vi "Begin.vi"(8 "error in":errorcluster) -> (0 "error out":errorcluster)   [LabVIEW 2018]
doc: "Called before other user functions, this VI is expected to open initial I/O refnums, load in file data, and do all program initialization. Notice that the <B>error out</B> terminal is simply used for data flow. Wiring it to other structures or subVIs ensures that this VI runs first."
uses:
  <vilib>/Rock Robotics/SystemInterfaces/DIO/FPGA_DIOPWMChannel.ctl
  <vilib>/Rock Robotics/WPI/DriverStation/WPI_DriverStationRobotMode2.ctl
  <vilib>/Rock Robotics/WPI/Joystick/WPI_JoystickDeviceEnum.ctl
  <vilib>/Rock Robotics/WPI/Solenoid/WPI_SolenoidChannel.ctl
  <vilib>/Rock Robotics/SystemInterfaces/DIO/FPGA_DIOChannel.ctl
  <vilib>/Rock Robotics/WPI/SafetyOutput/WPI_SafetyOutputConfigMenu.ctl
  Robot Global Data.vi
  <vilib>/Rock Robotics/Network Tables/NT Write String Array.vi
  <vilib>/Rock Robotics/WPI/RobotDrive/WPI_RobotDriveOpen4MotorWithTalonSRX.vi
  <vilib>/Rock Robotics/WPI/Switch/WPI_SwitchOpenLimit.vi
  <vilib>/Rock Robotics/WPI/MotorControl/WPI_MotorControlOpen TalonSRX.vi
  Global 1.vi
  <vilib>/Rock Robotics/WPI/Counter/WPI_CounterDigitalInputToDigitalSource.vi
  <vilib>/Rock Robotics/WPI/Solenoid/WPI_SolenoidOpenDouble.vi
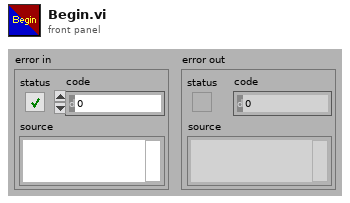
[diagram p1: front panel]
types:
  T1 = typedef "FPGA_DIOChannel.ctl" = enum8{"DIO 0", "DIO 1", "DIO 2", "DIO 3", "DIO 4", "DIO 5", "DIO 6", "DIO 7", "DIO 8", "DIO 9", "DIO MXP 0", "DIO MXP 1", "DIO MXP 2", "DIO MXP 3", "DIO MXP 4", "DIO MXP 5", "DIO MXP 6", "DIO MXP 7", "DIO MXP 8", "DIO MXP 9", "DIO MXP 10", "DIO MXP 11", "DIO MXP 12", "DIO MXP 13", "DIO MXP 14", "DIO MXP 15", "SPI Port CS1", "SPI Port CS2", "SPI Port CS3", "SPI Port MISO", "SPI Port MOSI", "Invalid"}
  T2 = typedef "WPI_SafetyOutputConfigMenu.ctl" = enum16{"Enable", "Disable"}
  T3 = typedef "FPGA_DIOPWMChannel.ctl" = enum8{"PWM 0", "PWM 1", "PWM 2", "PWM 3", "PWM 4", "PWM 5", "PWM 6", "PWM 7", "PWM 8", "PWM 9", "PWM MXP 0", "PWM MXP 1", "PWM MXP 2", "PWM MXP 3", "PWM MXP 4", "PWM MXP 5", "PWM MXP 6", "PWM MXP 7", "PWM MXP 8", "PWM MXP 9", "Invalid"}
  T4 = typedef "WPI_JoystickDeviceEnum.ctl" = enum16{"USB 0", "USB 1", "USB 2", "USB 3", "USB 4", "USB 5"}
  T5 = typedef "WPI_SolenoidChannel.ctl" = enum8{"Solenoid 0", "Solenoid 1", "Solenoid 2", "Solenoid 3", "Solenoid 4", "Solenoid 5", "Solenoid 6", "Solenoid 7", "Invalid"}
  T6 = typedef "WPI_DriverStationRobotMode2.ctl" = enum16{"Autonomous Disabled", "Autonomous Enabled", "Teleop Disabled", "Teleop Enabled", "Disconnected", "Finish", "Test Disabled", "Test Enabled", "Emergency Stopped"}
  T7 = typedef "WPI_MotorControlDeviceRef.ctl" = cluster{"DeviceStatus":errorcluster, "Type":T8, "PWM":cluster{"PWM Channel":T3, "DeadBand":T9}, "CAN":cluster{"Device Number":u8, "SetOutput VI Ref":variant, "GetOutput VI Ref":variant, "Enable VI Ref":variant, "Disable VI Ref":variant, "Data":variant}, "Invert":bool, "DIO PWM":cluster{"PWM \"Enable\" Channel":T3, "DIOChannel":T1, "PWM Rate":dbl}}
  T8 = typedef "WPI_MotorControlType.ctl" = enum16{"PWM", "CAN", "DIO PWM"}
  T9 = typedef "WPI_PWMDeadband.ctl" = cluster{"Name":string, "maxPositivePwm":i32, "minPositivePwm":i32, "centerPwm":i32, "maxNegativePwm":i32, "minNegativePwm":i32, "angularRange":u16}
  T10 = typedef "WPI_RobotDriveDevRef.ctl" = cluster{"DevStatus":errorcluster, "Motors[]":T7[], "Square Inputs":bool, "Max Output":dbl}
  T11 = typedef "WPI_JoystickDevRef.ctl" = cluster{"Device":T4}
  T12 = typedef "WPI_DigitalInputDevRef.ctl" = cluster{"DevStatus":errorcluster, "DIO Channel":T1}
  T13 = typedef "FPGA_CounterEncoderSourceConvertionLVSourceType.ctl" = cluster{"DevStatus":errorcluster, "AnalogTriggerMode?":bool, "DigitalMode":cluster{"DIO Channel":T14}, "AnalogTriggerMode":cluster{"AnalogTriggerIndex":T15, "OutputType":T16}}
  T14 = typedef "FPGA_DIODigitalSourceChannel.ctl" = enum8{"DIO 0", "DIO 1", "DIO 2", "DIO 3", "DIO 4", "DIO 5", "DIO 6", "DIO 7", "DIO 8", "DIO 9", "DIO MXP 0", "DIO MXP 1", "DIO MXP 2", "DIO MXP 3", "DIO MXP 4", "DIO MXP 5", "DIO MXP 6", "DIO MXP 7", "DIO MXP 8", "DIO MXP 9", "DIO MXP 10", "DIO MXP 11", "DIO MXP 12", "DIO MXP 13", "DIO MXP 14", "DIO MXP 15", "SPI Port CS1", "SPI Port CS2", "SPI Port CS3", "SPI Port MISO", "SPI Port MOSI", "Disabled"}
  T15 = typedef "FPGA_AnalogTriggerIndex.ctl" = enum8{"Trig 0", "Trig 1", "Trig 2", "Trig 3", "Trig 4", "Trig 5", "Trig 6", "Trig 7", "Invalid"}
  T16 = typedef "FPGA_AnalogTriggerOutType.ctl" = enum16{"InWindow", "TriggerState", "Rising", "Falling"}
  T17 = typedef "WPI_SolenoidDevRef.ctl" = cluster{"DevStatus":errorcluster, "Pneumatics Control Module":u8, "Forward Solenoid Channel":T5, "Reverse Solenoid Channel":T5}
  T18 = typedef "WPI_EncoderDevRef.ctl" = cluster{"DevStatus":errorcluster, "EncoderIndex":T19, "CounterIndex":T20, "DistancePerCount":dbl, "Decoding Type":T21}
  T19 = typedef "FPGA_EncoderIdx.ctl" = enum8{"Enc 0", "Enc 1", "Enc 2", "Enc 3", "Enc 4", "Enc 5", "Enc 6", "Enc 7", "Invalid"}
  T20 = typedef "FPGA_CounterCtrSystemIndex.ctl" = enum8{"Ctr 0", "Ctr 1", "Ctr 2", "Ctr 3", "Ctr 4", "Ctr 5", "Ctr 6", "Ctr 7", "Invalid"}
  T21 = typedef "WPI_EncoderType.ctl" = enum16{"1x", "2x", "4x"}
  T22 = typedef "WPI_SwitchDevRef.ctl" = cluster{"DevStatus":errorcluster, "DIO Channel":T1, "CntIndex":T20, "Normally Closed":bool}
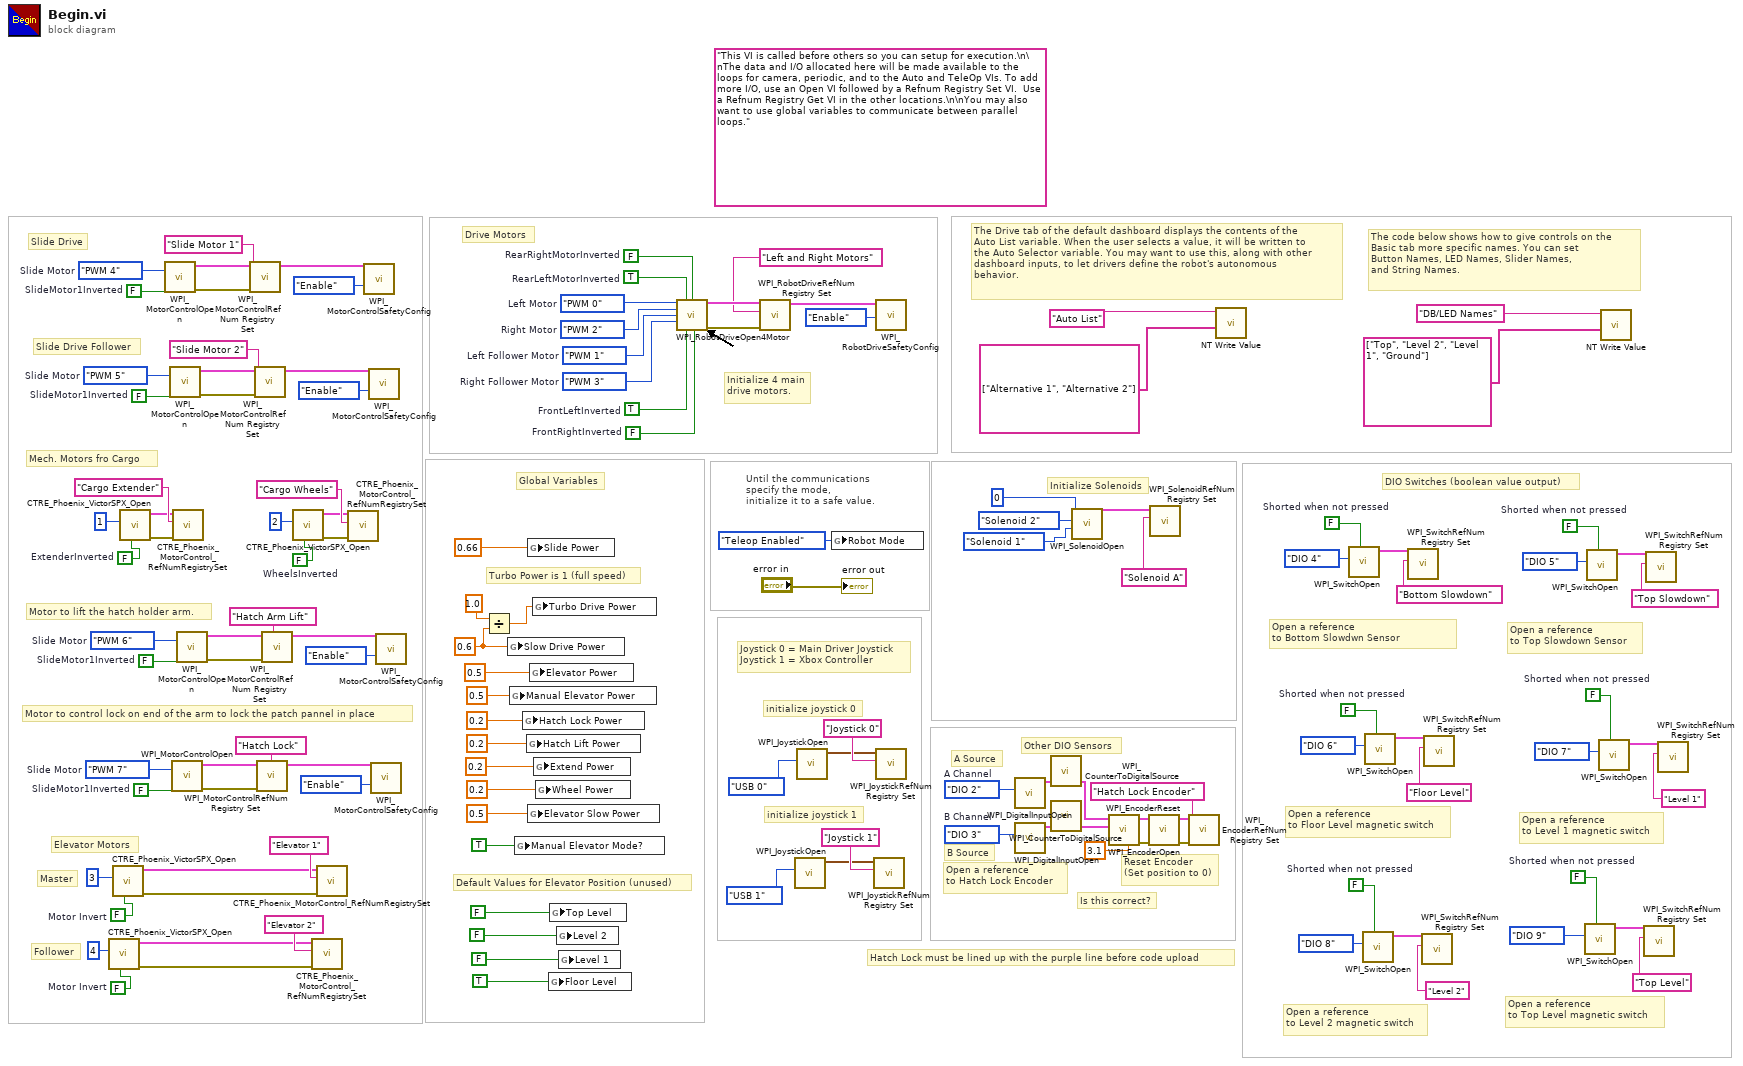
[diagram p0: block diagram]
diagram:
  w30 = FPGA_DIOChannel."DIO 3"  # B Channel
  w29 = FPGA_DIOChannel."DIO 2"  # A Channel
  w32 = FALSE  # Shorted when not pressed
  w36 = FALSE  # Shorted when not pressed
  w42 = FALSE  # SlideMotor1Inverted
  w47 = FPGA_DIOPWMChannel."PWM 7"  # Slide Motor
  w49 = FALSE  # SlideMotor1Inverted
  w54 = FPGA_DIOPWMChannel."PWM 6"  # Slide Motor
  w12 = FALSE  # Motor Invert
  w65 = FALSE  # SlideMotor1Inverted
  w71 = FPGA_DIOPWMChannel."PWM 5"  # Slide Motor
  w64 = FALSE  # WheelsInverted
  w60 = FALSE  # ExtenderInverted
  w4 = 0.6
  w55 = FALSE  # Motor Invert
  w81 = FALSE  # Shorted when not pressed
  w84 = FALSE  # SlideMotor1Inverted
  w90 = FPGA_DIOPWMChannel."PWM 4"  # Slide Motor
  w93 = FALSE  # Shorted when not pressed
  w94 = FALSE  # Shorted when not pressed
  w95 = FALSE  # Shorted when not pressed
  w109 = TRUE  # FrontLeftInverted
  w110 = FALSE  # FrontRightInverted
  w111 = FPGA_DIOPWMChannel."PWM 3"  # Right Follower Motor
  w112 = FPGA_DIOPWMChannel."PWM 1"  # Left Follower Motor
  (unwired) "This VI is called before others so you can setup for execution.\n\nThe data and I/O allocated here will be made available to the loops for camera, periodic, and to the Auto and TeleOp VIs. To add more I/O, use an Open VI followed by a Refnum Registry Set VI.  Use a Refnum Registry Get VI in the other locations.\n\nYou may also want to use global variables to communicate between parallel loops."
  w124 = FPGA_DIOPWMChannel."PWM 2"  # Right Motor
  w125 = FPGA_DIOPWMChannel."PWM 0"  # Left Motor
  w129 = TRUE  # RearLeftMotorInverted
  w130 = FALSE  # RearRightMotorInverted
  # "Turbo Power is 1 (full speed)"
  # "B Source"
  # "A Source"
  # "Hatch Lock must be lined up with the purple line before code upload"
  # "Is this correct?"
  # "Reset Encoder\n(Set position to 0)"
  # "Open a reference\nto Hatch Lock Encoder"
  # "Other DIO Sensors"
  # "DIO Switches (boolean value output)"
  # "Open a reference\nto Top Slowdown Sensor"
  # "Open a reference\nto Bottom Slowdwn Sensor"
  # "Default Values for Elevator Position (unused)"
  # "Elevator Motors"
  # "Motor to control lock on end of the arm to lock the patch pannel in place"
  # "Motor to lift the hatch holder arm."
  # "Global Variables"
  # "Follower"
  # "Master"
  # "Slide Drive Follower"
  # "Slide Drive"
  # "Open a reference\nto Top Level magnetic switch"
  # "Drive Motors"
  # "Mech. Motors fro Cargo"
  # "Open a reference\nto Level 2 magnetic switch"
  # "Open a reference\nto Level 1 magnetic switch"
  # "Open a reference\nto Floor Level magnetic switch"
  # "Initialize Solenoids"
  # "Initialize 4 main\ndrive motors."
  # "Joystick 0 = Main Driver Joystick\nJoystick 1 = Xbox Controller"
  # "initialize joystick 1"
  # "The Drive tab of the default dashboard displays the contents of the\nAuto List variable. When the user selects a value, it will be written to\nthe Auto Selector variable. You may want to use this, along with other\ndashboard inputs, to let drivers define the robot's autonomous\nbehavior."
  # "The code below shows how to give controls on the\nBasic tab more specific names. You can set\nButton Names, LED Names, Slider Names,\nand String Names."
  # "initialize joystick 0"
  # "Until the communications \nspecify the mode,\ninitialize it to a safe value."
  n1 = call <vilib>:"CTRE_Phoenix_VictorSPX_Open.vi"("Invert"=w12, "Device Number"=u8 4) -> ("error out"=w15:errorcluster, "CAN Talon SRX Ref"=w14:T7)  [unwired: 8 in]
  n2 = call <vilib>:"CTRE_Phoenix_VictorSPX_Open.vi"("Invert"=w55, "Device Number"=u8 3) -> ("error out"=w16:errorcluster, "CAN Talon SRX Ref"=w17:T7)  [unwired: 8 in]
  n3 = call <vilib>:"CTRE_Phoenix_VictorSPX_Open.vi"("Invert"=w60, "Device Number"=u8 1) -> ("error out"=w57:errorcluster, "CAN Talon SRX Ref"=w58:T7)  [unwired: 8 in]
  n4 = call-poly <vilib>:"WPI_MotorControlOpen.vi"("Invert"=w84, "PWM Channel"=w90) -> ("error out"=w88:errorcluster, "MotorControlDeviceRef"=w89:T7)  [unwired: 8 in]
  n5 = call-poly <vilib>:"WPI_MotorControlOpen.vi"("Invert"=w65, "PWM Channel"=w71) -> ("error out"=w69:errorcluster, "MotorControlDeviceRef"=w70:T7)  [unwired: 8 in]
  n6 = call-poly <vilib>:"WPI_MotorControlOpen.vi"("Invert"=w42, "PWM Channel"=w47) -> ("error out"=w45:errorcluster, "MotorControlDeviceRef"=w46:T7)  [unwired: 8 in]
  n7 = call <vilib>:"CTRE_Phoenix_MotorControl_RefNumRegistrySet.vi"("error in (no error)"=w57, "refnum name"="Cargo Extender", "PhoenixMotorControlDevRef"=w58) -> ()  [unwired: 7 in, 2 out]
  n8 = call-poly <vilib>:"WPI_MotorControlOpen.vi"("Invert"=w49, "PWM Channel"=w54) -> ("error out"=w52:errorcluster, "MotorControlDeviceRef"=w53:T7)  [unwired: 8 in]
  n9 = call <vilib>:"WPI_MotorControlRefNum Registry Set.vi"("error in (no error)"=w88, "refnum name"="Slide Motor 1", "MotorControlDevRef"=w89) -> ("MotorControlDevRef"=w86:T7)  [unwired: 7 in, 1 out]
  n10 = call <vilib>:"WPI_MotorControlRefNum Registry Set.vi"("error in (no error)"=w69, "refnum name"="Slide Motor 2", "MotorControlDevRef"=w70) -> ("MotorControlDevRef"=w67:T7)  [unwired: 7 in, 1 out]
  n11 = call <vilib>:"WPI_MotorControlRefNum Registry Set.vi"("error in (no error)"=w45, "refnum name"="Hatch Lock", "MotorControlDevRef"=w46) -> ("MotorControlDevRef"=w44:T7)  [unwired: 7 in, 1 out]
  n12 = call <vilib>:"WPI_MotorControlRefNum Registry Set.vi"("error in (no error)"=w52, "refnum name"="Hatch Arm Lift", "MotorControlDevRef"=w53) -> ("MotorControlDevRef"=w51:T7)  [unwired: 7 in, 1 out]
  n13 = call <vilib>:"CTRE_Phoenix_VictorSPX_Open.vi"("Invert"=w64, "Device Number"=u8 2) -> ("error out"=w61:errorcluster, "CAN Talon SRX Ref"=w62:T7)  [unwired: 8 in]
  n14 = call <vilib>:"CTRE_Phoenix_MotorControl_RefNumRegistrySet.vi"("error in (no error)"=w15, "refnum name"="Elevator 2", "PhoenixMotorControlDevRef"=w14) -> ()  [unwired: 7 in, 2 out]
  n15 = call <vilib>:"CTRE_Phoenix_MotorControl_RefNumRegistrySet.vi"("error in (no error)"=w16, "refnum name"="Elevator 1", "PhoenixMotorControlDevRef"=w17) -> ()  [unwired: 7 in, 2 out]
  n16 = call <vilib>:"CTRE_Phoenix_MotorControl_RefNumRegistrySet.vi"("error in (no error)"=w61, "refnum name"="Cargo Wheels", "PhoenixMotorControlDevRef"=w62) -> ()  [unwired: 7 in, 2 out]
  n17 = call <vilib>:"WPI_MotorControlSafetyConfig.vi"("mode"=WPI_SafetyOutputConfigMenu."Enable", "MotorControlDevRef"=w86) -> ()  [unwired: 8 in, 2 out]
  n18 = call <vilib>:"WPI_MotorControlSafetyConfig.vi"("mode"=WPI_SafetyOutputConfigMenu."Enable", "MotorControlDevRef"=w67) -> ()  [unwired: 8 in, 2 out]
  n19 = call <vilib>:"WPI_MotorControlSafetyConfig.vi"("mode"=WPI_SafetyOutputConfigMenu."Enable", "MotorControlDevRef"=w44) -> ()  [unwired: 8 in, 2 out]
  n20 = call <vilib>:"WPI_MotorControlSafetyConfig.vi"("mode"=WPI_SafetyOutputConfigMenu."Enable", "MotorControlDevRef"=w51) -> ()  [unwired: 8 in, 2 out]
  n21 = Divide(x=1.0, y=w4) -> (x/y=w3:dbl)
  n22 = global write "Global 1.vi" "Slow Drive Power"(w4) -> ()
  n23 = global write "Global 1.vi" "Manual Elevator Power"(0.5) -> ()
  n24 = global write "Global 1.vi" "Manual Elevator Mode?"(TRUE) -> ()
  n25 = global write "Global 1.vi" "Hatch Lock Power"(0.2) -> ()
  n26 = global write "Global 1.vi" "Hatch Lift Power"(0.2) -> ()
  n27 = global write "Global 1.vi" "Slide Power"(0.66) -> ()
  n28 = global write "Global 1.vi" "Elevator Slow Power"(0.5) -> ()
  n29 = global write "Global 1.vi" "Elevator Power"(0.5) -> ()
  n30 = global write "Global 1.vi" "Turbo Drive Power"(w3) -> ()
  n31 = global write "Global 1.vi" "Extend Power"(0.2) -> ()
  n32 = global write "Global 1.vi" "Wheel Power"(0.2) -> ()
  n33 = global write "Global 1.vi" "Floor Level"(TRUE) -> ()
  n34 = global write "Global 1.vi" "Top Level"(FALSE) -> ()
  n35 = global write "Global 1.vi" "Level 2"(FALSE) -> ()
  n36 = global write "Global 1.vi" "Level 1"(FALSE) -> ()
  n37 = call-poly <vilib>:"WPI_RobotDriveOpen4Motor.vi"("Rear Left Motor"=w125, "Rear Left Motor Inverted"=w129, "Rear Right Motor Inverted"=w130, "Rear Right Motor"=w124, "Front Left Motor"=w112, "Front Right Motor"=w111, "Front Left Motor Inverted"=w109, "Front Right Motor Inverted"=w110) -> ("RobotDriveDevRef"=w128:T10, "error out"=w126:errorcluster)  [unwired: 6 in]
  n38 = call <vilib>:"WPI_RobotDriveRefNum Registry Set.vi"("error in (no error)"=w126, "refnum name"="Left and Right Motors", "RobotDriveDevRef"=w128) -> ("RobotDriveDevRef"=w123:T10)  [unwired: 1 in, 7 out]
  n39 = call <vilib>:"WPI_JoystickOpen.vi"("JoystickDevice"=WPI_JoystickDeviceEnum."USB 1") -> ("JoystickDevRef"=w104:T11)  [unwired: 10 in]
  n40 = call <vilib>:"WPI_JoystickOpen.vi"("JoystickDevice"=WPI_JoystickDeviceEnum."USB 0") -> ("JoystickDevRef"=w119:T11)  [unwired: 10 in]
  n41 = global write "Robot Global Data.vi" "Robot Mode"(WPI_DriverStationRobotMode2."Teleop Enabled" ("Robot Mode")) -> ()
  n42 = call <vilib>:"WPI_JoystickRefNum Registry Set.vi"("refnum name"="Joystick 1", "JoystickDevRef"=w104) -> ()  [unwired: 8 in, 2 out]
  n43 = call <vilib>:"WPI_RobotDriveSafetyConfig.vi"("mode"=WPI_SafetyOutputConfigMenu."Enable", "RobotDriveDevRef"=w123) -> ()  [unwired: 8 in, 2 out]
  n44 = call <vilib>:"WPI_JoystickRefNum Registry Set.vi"("refnum name"="Joystick 0", "JoystickDevRef"=w119) -> ()  [unwired: 8 in, 2 out]
  n45 = call <vilib>:"WPI_DigitalInputOpen.vi"("DIO Channel"=w29) -> ("DigitalInputDevRef"=w26:T12)  [unwired: 1 in, 9 out]
  n46 = call <vilib>:"WPI_DigitalInputOpen.vi"("DIO Channel"=w30) -> ("DigitalInputDevRef"=w27:T12)  [unwired: 1 in, 9 out]
  n47 = call-poly <vilib>:"WPI_CounterToDigitalSource.vi"("DigitalInputDevRef"=w26) -> ("Digital Source"=w25:T13)  [unwired: 6 out]
  n48 = call-poly <vilib>:"WPI_CounterToDigitalSource.vi"("DigitalInputDevRef"=w27) -> ("Digital Source"=w28:T13)  [unwired: 6 out]
  n49 = call-poly <vilib>:"WPI_SolenoidOpen.vi"("Reverse Solenoid Channel"=WPI_SolenoidChannel."Solenoid 1" ("Solenoid Channel"), "Forward Solenoid Channel"=WPI_SolenoidChannel."Solenoid 2" ("Solenoid Channel"), "Pneumatics Control Module (0)"=u8 0) -> ("SolenoidDevRef"=w107:T17)  [unwired: 7 in, 1 out]
  n50 = call <vilib>:"WPI_EncoderOpen.vi"("DistancePerCount"=3.1, "BSource"=w28, "ASource"=w25) -> ("error out"=w22:errorcluster, "EncoderDevRef"=w21:T18)  [unwired: 5 in, 2 out]
  n51 = call <vilib>:"WPI_EncoderReset.vi"("error in (no error)"=w22, "EncoderDevRef"=w21) -> ("error out"=w19:errorcluster, "EncoderDevRef"=w20:T18)  [unwired: 8 in]
  n52 = call <vilib>:"WPI_SolenoidRefNum Registry Set.vi"("refnum name"="Solenoid A", "SolenoidDevRef"=w107) -> ()  [unwired: 8 in, 2 out]
  n53 = call <vilib>:"WPI_EncoderRefNum Registry Set.vi"("error in (no error)"=w19, "refnum name"="Hatch Lock Encoder", "EncoderDevRef"=w20) -> ()  [unwired: 7 in, 2 out]
  n54 = call-poly <vilib>:"NT Write Value.vi"("String Array"=string[] ["Alternative 1", "Alternative 2"], "Name"="Auto List") -> ()  [unwired: 9 in, 1 out]
  n55 = call-poly <vilib>:"WPI_SwitchOpen.vi"("Normally Closed"=w36, "DIO Channel"=FPGA_DIOChannel."DIO 4") -> ("SwitchDevRef"=w39:T22)  [unwired: 8 in, 1 out]
  n56 = call-poly <vilib>:"WPI_SwitchOpen.vi"("Normally Closed"=w93, "DIO Channel"=FPGA_DIOChannel."DIO 8") -> ("SwitchDevRef"=w98:T22)  [unwired: 8 in, 1 out]
  n57 = call-poly <vilib>:"WPI_SwitchOpen.vi"("Normally Closed"=w95, "DIO Channel"=FPGA_DIOChannel."DIO 6") -> ("SwitchDevRef"=w102:T22)  [unwired: 8 in, 1 out]
  n58 = call <vilib>:"WPI_SwitchRefNum Registry Set.vi"("refnum name"="Bottom Slowdown", "SwitchDevRef"=w39) -> ()  [unwired: 8 in, 2 out]
  n59 = call <vilib>:"WPI_SwitchRefNum Registry Set.vi"("refnum name"="Level 2", "SwitchDevRef"=w98) -> ()  [unwired: 8 in, 2 out]
  n60 = call <vilib>:"WPI_SwitchRefNum Registry Set.vi"("refnum name"="Floor Level", "SwitchDevRef"=w102) -> ()  [unwired: 8 in, 2 out]
  n61 = call-poly <vilib>:"WPI_SwitchOpen.vi"("Normally Closed"=w81, "DIO Channel"=FPGA_DIOChannel."DIO 9") -> ("SwitchDevRef"=w83:T22)  [unwired: 8 in, 1 out]
  n62 = call-poly <vilib>:"WPI_SwitchOpen.vi"("Normally Closed"=w32, "DIO Channel"=FPGA_DIOChannel."DIO 5") -> ("SwitchDevRef"=w35:T22)  [unwired: 8 in, 1 out]
  n63 = call-poly <vilib>:"WPI_SwitchOpen.vi"("Normally Closed"=w94, "DIO Channel"=FPGA_DIOChannel."DIO 7") -> ("SwitchDevRef"=w100:T22)  [unwired: 8 in, 1 out]
  n64 = call-poly <vilib>:"NT Write Value.vi"("String Array"=string[] ["Top", "Level 2", "Level 1", "Ground"], "Name"="DB/LED Names") -> ()  [unwired: 9 in, 1 out]
  n65 = call <vilib>:"WPI_SwitchRefNum Registry Set.vi"("refnum name"="Top Level", "SwitchDevRef"=w83) -> ()  [unwired: 8 in, 2 out]
  n66 = call <vilib>:"WPI_SwitchRefNum Registry Set.vi"("refnum name"="Top Slowdown", "SwitchDevRef"=w35) -> ()  [unwired: 8 in, 2 out]
  n67 = call <vilib>:"WPI_SwitchRefNum Registry Set.vi"("refnum name"="Level 1", "SwitchDevRef"=w100) -> ()  [unwired: 8 in, 2 out]
  "error out" <- "error in"
